vi "Report Generator.vi"(8 "error in (no error)":errorcluster, 11 "Report Generator In":refnum<class "Report Generator.lvclass">) -> (0 "error out":errorcluster)   [LabVIEW 2020, in "Reports.lvlib" / "Report Generator.lvclass"]
uses:
  Report Generator.lvclass
  Report Generator.lvclass/Report Generator.ctl
  User Interface/Process/Process.lvclass
  User Interface/Error Handler/Error Handler.lvclass
  <vilib>/Platform/browser.llb/Open URL in Default Browser (path).vi
  Framework/Report Interface/Report Interface.lvclass
  C:/git/astemes-lunit/source/User Interface/Process/Process.lvclass
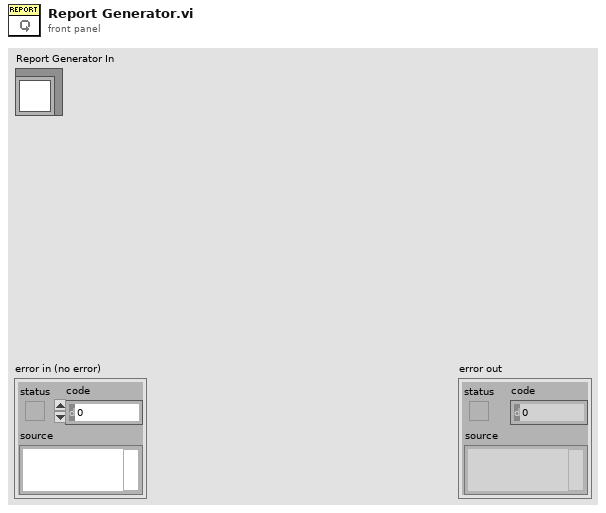
[diagram p1: front panel]
types:
  T1 = typedef "Result.lvlib/Result.ctl" = cluster{"Name":string, "Message":string, "Description":string, "Status":T2, "Result Type":T3, "Execution Time":dbl}
  T2 = typedef "Result.lvlib/Status.ctl" = enum16{"", "Passed", "Failed", "Error", "Skipped", "Setup Error", "Broken", "Teardown Error"}
  T3 = typedef "Result.lvlib/Type.ctl" = enum16{"Test Case", "Test Suite", "Test Run", "Pass", "Fail", "Skip", "Pass if", "Fail if", "Pass if Error", "Fail if Error", "Pass if Equal", "Fail if Equal"}
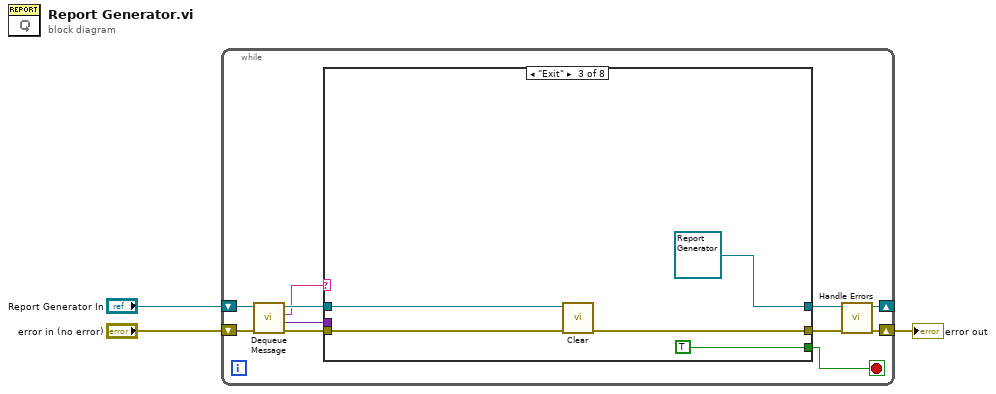
[diagram p0: block diagram]
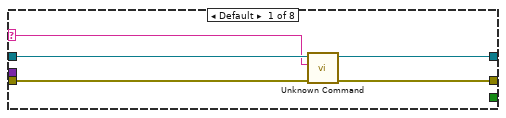
[diagram p2: hidden frame]
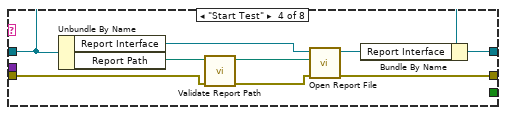
[diagram p4: hidden frame]
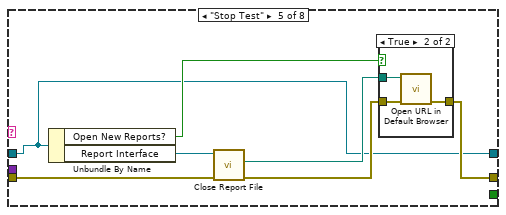
[diagram p5: hidden frame]
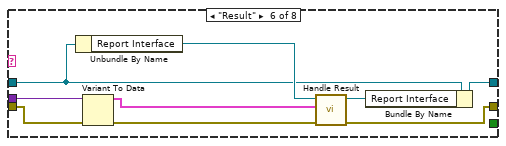
[diagram p7: hidden frame]
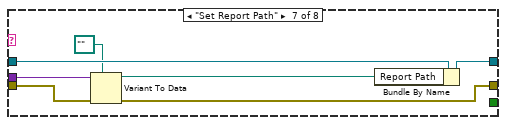
[diagram p8: hidden frame]
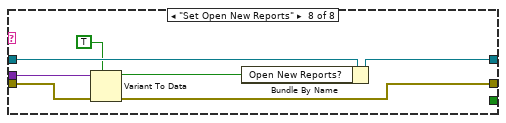
[diagram p9: hidden frame]
diagram:
  n1 = while {
    shift-right: [w6] -> w1
    shift-left: "error in (no error)" -> [w13]
    shift-right: [w8] -> _
    shift-left: "Report Generator In" -> [w11]
    stop <- w7 stop-if-true
    n2 = call "Dequeue Message.vi"("error in (no error)"=w13, "Process In"=w11) -> ("error out"=w12:errorcluster, "Message Data"=w10:variant, "Message"=w5:string, "Process Out"=w9:refnum<class "Report Generator.lvclass">)  [unwired: 6 in]
    n3 = case shown="\"Exit\"" w5 {
      selector: w5 -> [w14 _ _ _ _ _ _ _]
      tunnel: w12 -> [w18 w19 w23 w26 w41 w54 w61 w68]
      tunnel: [w17 w19 w22 w34 w39 w53 w56 w65] -> w4
      tunnel: w10 -> [_ _ _ _ _ w51 w58 w64]
      tunnel: w9 -> [w16 w20 w24 w30 w35 w47 w60 w67]
      tunnel: [w15 w20 refnum<class "Report Generator.lvclass"> refnum ("Process Out") w32 w35 w48 w59 w66] -> w8
      tunnel: [_ _ TRUE _ _ _ _ _] -> w7
      frame Default {
        n4 = call "Unknown Command.vi"("error in (no error)"=w18, "String"=w14, "Process In"=w16) -> ("error out"=w17:errorcluster, "Process Out"=w15:refnum<class "Report Generator.lvclass">)  [unwired: 7 in]
      }
      frame "Init" {
      }
      frame "Exit" {
        n5 = call-dynamic "Clear.vi"("error in (no error)"=w23, "Report Generator In"=w24) -> ("error out"=w22:errorcluster)  [unwired: 9 in]
      }
      frame "Start Test" {
        n6 = Unbundle By Name(w30) -> ("Report Interface"=w33:refnum<class "Report Interface.lvclass">, "Report Path"=w29:path)
        n7 = call "Validate Report Path.vi"("error in (no error)"=w26, "Path"=w29) -> ("error out"=w27:errorcluster, "path"=w28:path)  [unwired: 8 in]
        n8 = call-dynamic "Open Report File.vi"("error in (no error)"=w27, "Path"=w28, "Report Interface In"=w33) -> ("error out"=w34:errorcluster, "Report Interface Out"=w31:refnum<class "Report Interface.lvclass">)  [unwired: 7 in]
        n9 = Bundle By Name(cluster=w30, "Report Interface"=w31) -> (w32:refnum<class "Report Generator.lvclass">)
      }
      frame "Stop Test" {
        n10 = Unbundle By Name(w35) -> ("Open New Reports?"=w38:bool, "Report Interface"=w36:refnum<class "Report Interface.lvclass">)
        n11 = call-dynamic "Close Report File.vi"("error in (no error)"=w41, "Report Interface In"=w36) -> ("error out"=w40:errorcluster, "Report Path"=w37:path)  [unwired: 8 in]
        n12 = case shown="True" w38 {
          tunnel: w37 -> [_ w43]
          tunnel: w40 -> [w42 w45]
          tunnel: [w42 w44] -> w39
          frame False {
          }
          frame True {
            n13 = call-poly <vilib>:"Open URL in Default Browser.vi"("error in (no error)"=w45, "path"=w43) -> ("error out"=w44:errorcluster)  [unwired: 4 in, 1 out]
          }
        }
      }
      frame "Result" {
        n14 = Unbundle By Name(w47) -> ("Report Interface"=w49:refnum<class "Report Interface.lvclass">)
        n15 = Variant To Data(error in=w54, Variant=w51) -> (data=w50:T1, error out=w52:errorcluster)  [unwired: 1 in]
        n16 = call-dynamic "Handle Result.vi"("error in (no error)"=w52, "Result"=w50, "Report in"=w49) -> ("error out"=w53:errorcluster, "Report out"=w46:refnum<class "Report Interface.lvclass">)  [unwired: 7 in]
        n17 = Bundle By Name(cluster=w47, "Report Interface"=w46) -> (w48:refnum<class "Report Generator.lvclass">)
      }
      frame "Set Report Path" {
        n18 = Variant To Data(error in=w61, type=path "", Variant=w58) -> (data=w55:path, error out=w56:errorcluster)
        n19 = Bundle By Name(cluster=w60, "Report Path"=w55) -> (w59:refnum<class "Report Generator.lvclass">)
      }
      frame "Set Open New Reports" {
        n20 = Variant To Data(error in=w68, type=TRUE, Variant=w64) -> (data=w63:bool, error out=w65:errorcluster)
        n21 = Bundle By Name(cluster=w67, "Open New Reports?"=w63) -> (w66:refnum<class "Report Generator.lvclass">)
      }
    }
    n22 = call "Handle Errors.vi"("error in (no error)"=w4) -> ("error out"=w6:errorcluster)  [unwired: 10 in]
  }
  "error out" <- w1
